vi "Process Mouse Wheel Event.vi"(10 "Delta":i32, 11 "Core Data in":T1) -> (3 "Core Data out":T1)   [LabVIEW 2020, in "Example 1.lvlib"]
uses:
  Example 1.lvlib
  Scene/Scene.lvclass
  Core Data.ctl
  Scene/Mouse Button Held.ctl
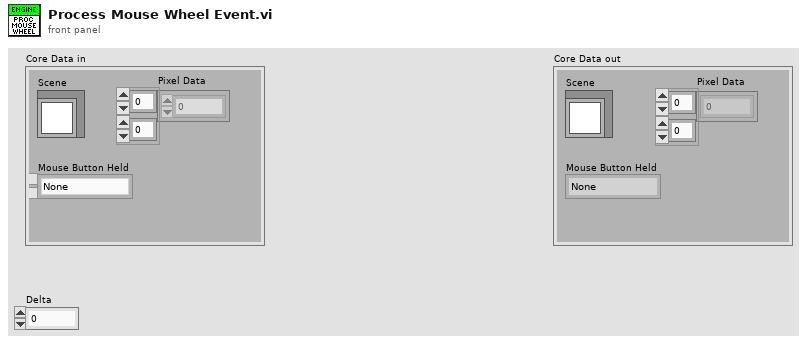
[diagram p1: front panel]
types:
  T1 = typedef "Example 1.lvlib/Core Data.ctl" = cluster{"Pixel Data":u32[][], "Scene":refnum<class "Scene.lvclass">, "Mouse Button Held":T2}
  T2 = typedef "Scene.lvclass/Mouse Button Held.ctl" = enum16{"None", "Left", "Middle", "Right"}
  T3 = typedef "3D.lvlib/Transform.ctl" = cluster{"Position":T4, "Rotation":T4, "Scale":T4}
  T4 = typedef "3D.lvlib/Vector 3D.ctl" = cluster{"x":sgl, "y":sgl, "z":sgl}
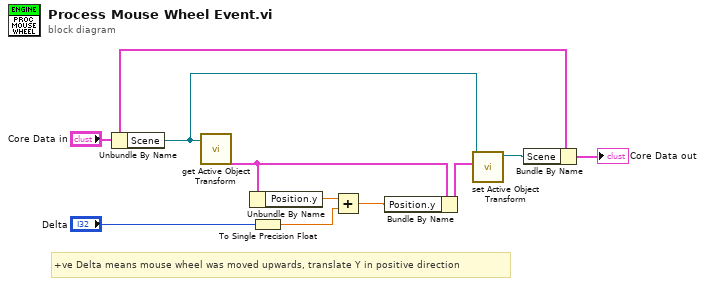
[diagram p0: block diagram]
diagram:
  # "+ve Delta means mouse wheel was moved upwards, translate Y in positive direction"
  n1 = Unbundle By Name("Core Data in") -> ("Scene"=w5:refnum<class "Scene.lvclass">)
  n2 = call "get Active Object Transform.vi"("Scene in"=w5) -> ("Transform"=w4:T3)  [unwired: 10 in]
  n3 = Unbundle By Name(w4) -> ("Position.y"=w8:sgl)
  n4 = To Single Precision Float(number="Delta") -> (single precision float=w1:sgl)
  n5 = Add(x=w8, y=w1) -> (x+y=w7:sgl)
  n6 = Bundle By Name(cluster=w4, "Position.y"=w7) -> (w3:T3)
  n7 = call "set Active Object Transform.vi"("Transform"=w3, "Scene in"=w5) -> ("Scene out"=w6:refnum<class "Scene.lvclass">)  [unwired: 9 in]
  n8 = Bundle By Name(cluster="Core Data in", "Scene"=w6) -> (→"Core Data out":T1)
